vi "Pin Toggle.vi"(8 "Error In":errorcluster) -> (0 "Error Out":errorcluster)   [LabVIEW 2014, in "STM32F4 Discovery General Wrapper.lvlib"]
uses:
  <vilib>/Aledyne-TSXperts/Arduino Compatible Compiler for LabVIEW/addons/STM32F4 Discovery General Wrapper/STM32F4 Discovery General Wrapper.lvlib
  <vilib>/Aledyne-TSXperts/Arduino Compatible Compiler for LabVIEW/addons/STM32F4 Discovery General Wrapper/Ctl/PinModes.ctl
  <vilib>/Aledyne-TSXperts/Arduino Compatible Compiler for LabVIEW/addons/STM32F4 Discovery General Wrapper/Ctl/PinList.ctl
  <vilib>/Aledyne-TSXperts/Arduino Compatible Compiler for LabVIEW/Arduino Compatible Compiler for LabVIEW.lvlib
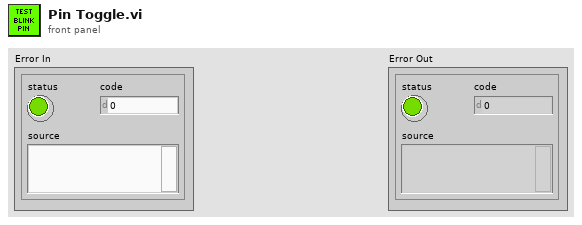
[diagram p1: front panel]
types:
  T1 = typedef "STM32F4 Discovery General Wrapper.lvlib/PinList.ctl" = enum8{"PA0", "PA1", "PA2", "PA3", "PA4", "PA5", "PA6", "PA7", "PA8", "PA9", "PA10", "PA11", "PA12", "PA13", "PA14", "PA15", "PB0", "PB1", "PB2", "PB3", "PB4", "PB5", "PB6", "PB7", "PB8", "PB9", "PB10", "PB11", "PB12", "PB13", "PB14", "PB15", "PC0", "PC1", "PC2", "PC3", "PC4", "PC5", "PC6", "PC7", "PC8", "PC9", "PC10", "PC11", "PC12", "PC13", "PC14", "PC15", "PD0", "PD1", "PD2", "PD3", "PD4", "PD5", "PD6", "PD7", "PD8", "PD9", "PD10", "PD11", "PD12", "PD13", "PD14", "PD15", "PE0", "PE1", "PE2", "PE3", "PE4", "PE5", "PE6", "PE7", "PE8", "PE9", "PE10", "PE11", "PE12", "PE13", "PE14", "PE15", "PF0", "PF1", "PF2", "PF3", "PF4", "PF5", "PF6", "PF7", "PF8", "PF9", "PF10", "PF11", "PF12", "PF13", "PF14", "PF15", "PG0", "PG1", "PG2", "PG3", "PG4", "PG5", "PG6", "PG7", "PG8", "PG9", "PG10", "PG11", "PG12", "PG13", "PG14", "PG15"}
  T2 = typedef "STM32F4 Discovery General Wrapper.lvlib/PinModes.ctl" = enum16{"OUTPUT", "OUTPUT_OPEN_DRAIN", "INPUT", "INPUT_ANALOG", "INPUT_PULLUP", "INPUT_PULLDOWN", "INPUT_FLOATING", "PWM", "PWM_OPEN_DRAIN"}
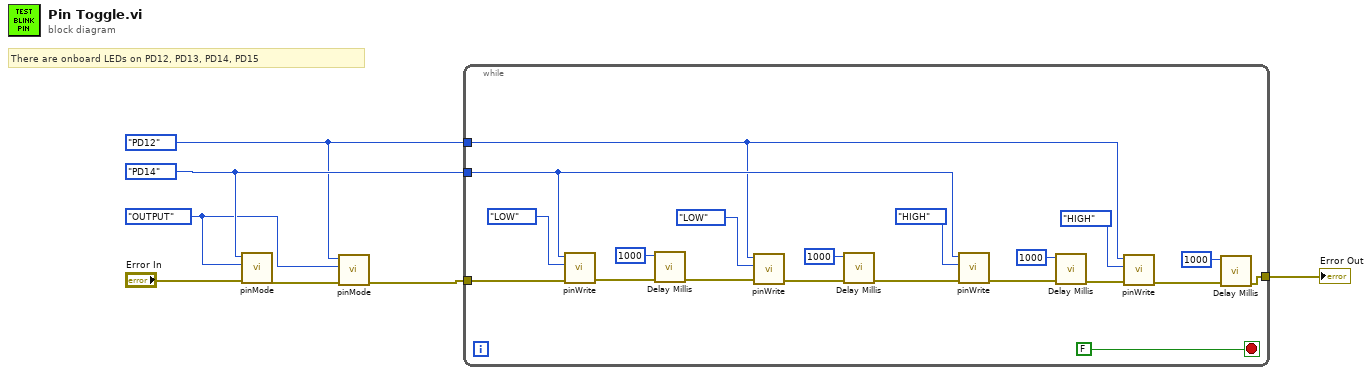
[diagram p0: block diagram]
diagram:
  w1 = PinList."PD12" ("Pin number")
  w5 = PinList."PD14" ("Pin number")
  w2 = PinModes."OUTPUT" ("Pin mode")
  # "There are onboard LEDs on PD12, PD13, PD14, PD15"
  n1 = call <vilib>:"pinMode.vi"("Error In"="Error In", "Pin mode"=w2, "Pin number"=w5) -> ("Error Out"=w3:errorcluster)  [unwired: 8 in]
  n2 = call <vilib>:"pinMode.vi"("Error In"=w3, "Pin mode"=w2, "Pin number"=w1) -> ("Error Out"=w4:errorcluster)  [unwired: 8 in]
  n3 = while {
    tunnel: w5 -> [w25]
    tunnel: [w8] -> w6
    tunnel: w4 -> [w19]
    tunnel: w1 -> [w9]
    stop <- FALSE stop-if-true
    n4 = call <vilib>:"pinWrite.vi"("Error In"=w19, "State 2"=enum16{"LOW", "HIGH"}."LOW", "Pin number"=w25) -> ("Error Out"=w23:errorcluster)  [unwired: 8 in]
    n5 = call <vilib>:"Delay Millis.vi"("error in (no error)"=w23, "delay"=u32 1000) -> ("error out"=w15:errorcluster)  [unwired: 9 in]
    n6 = call <vilib>:"pinWrite.vi"("Error In"=w15, "State 2"=enum16{"LOW", "HIGH"}."LOW", "Pin number"=w9) -> ("Error Out"=w17:errorcluster)  [unwired: 8 in]
    n7 = call <vilib>:"Delay Millis.vi"("error in (no error)"=w17, "delay"=u32 1000) -> ("error out"=w14:errorcluster)  [unwired: 9 in]
    n8 = call <vilib>:"pinWrite.vi"("Error In"=w14, "State 2"=enum16{"LOW", "HIGH"}."HIGH", "Pin number"=w25) -> ("Error Out"=w20:errorcluster)  [unwired: 8 in]
    n9 = call <vilib>:"Delay Millis.vi"("error in (no error)"=w20, "delay"=u32 1000) -> ("error out"=w10:errorcluster)  [unwired: 9 in]
    n10 = call <vilib>:"pinWrite.vi"("Error In"=w10, "State 2"=enum16{"LOW", "HIGH"}."HIGH", "Pin number"=w9) -> ("Error Out"=w13:errorcluster)  [unwired: 8 in]
    n11 = call <vilib>:"Delay Millis.vi"("error in (no error)"=w13, "delay"=u32 1000) -> ("error out"=w8:errorcluster)  [unwired: 9 in]
  }
  "Error Out" <- w6
